vi "MeasurePower.vi"(0 "object in":refnum<class "InstrumentBase.lvclass">, 5 "error in (no error)":errorcluster) -> (14 "object out":refnum<class "InstrumentBase.lvclass">, 16 "Measured Power":dbl, 17 "Channels array":waveform(dbl)[](array[waveform]), 19 "error out":errorcluster)   [LabVIEW 2019, in "InstrumentBase.lvclass"]
uses:
  InstrumentBase.lvclass
  InstrumentBase.lvclass/InstrumentBase.ctl
  <vilib>/Analysis/baseanly.llb/Mean (DBL).vi
  <vilib>/measure/matone.llb/Extract Single Tone Information 1 Chan.vi
  <vilib>/measure/madcrms.llb/Basic Averaged DC-RMS for 1 Chan.vi
  <vilib>/measure/NI_MAPro.lvlib
  <vilib>/Analysis/NI_AALBase.lvlib
panel:
  out "MeasuredPower4":dbl
  out "MeasuredPower3":dbl
  out "Measured Power 2":dbl
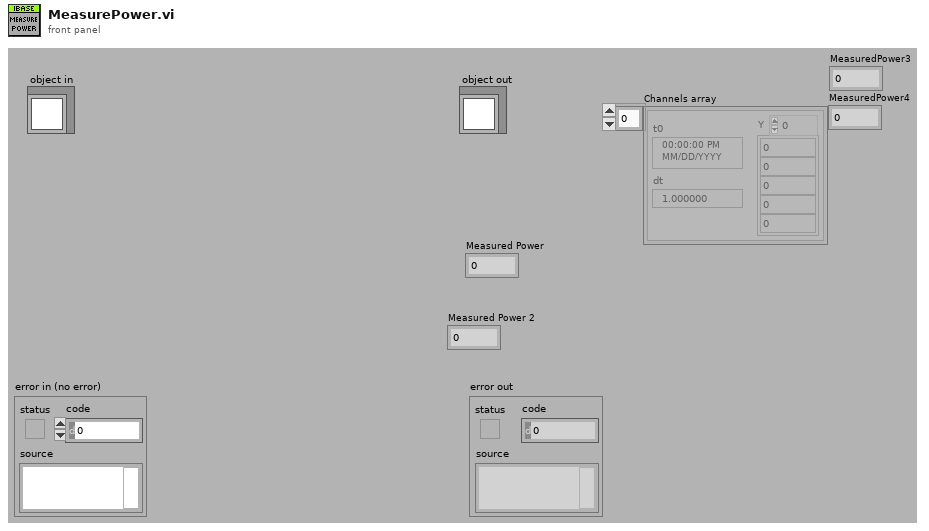
[diagram p1: front panel]
types:
  T1 = enum16{"Rectangular (none)", "Hanning", "Low side lobe"}
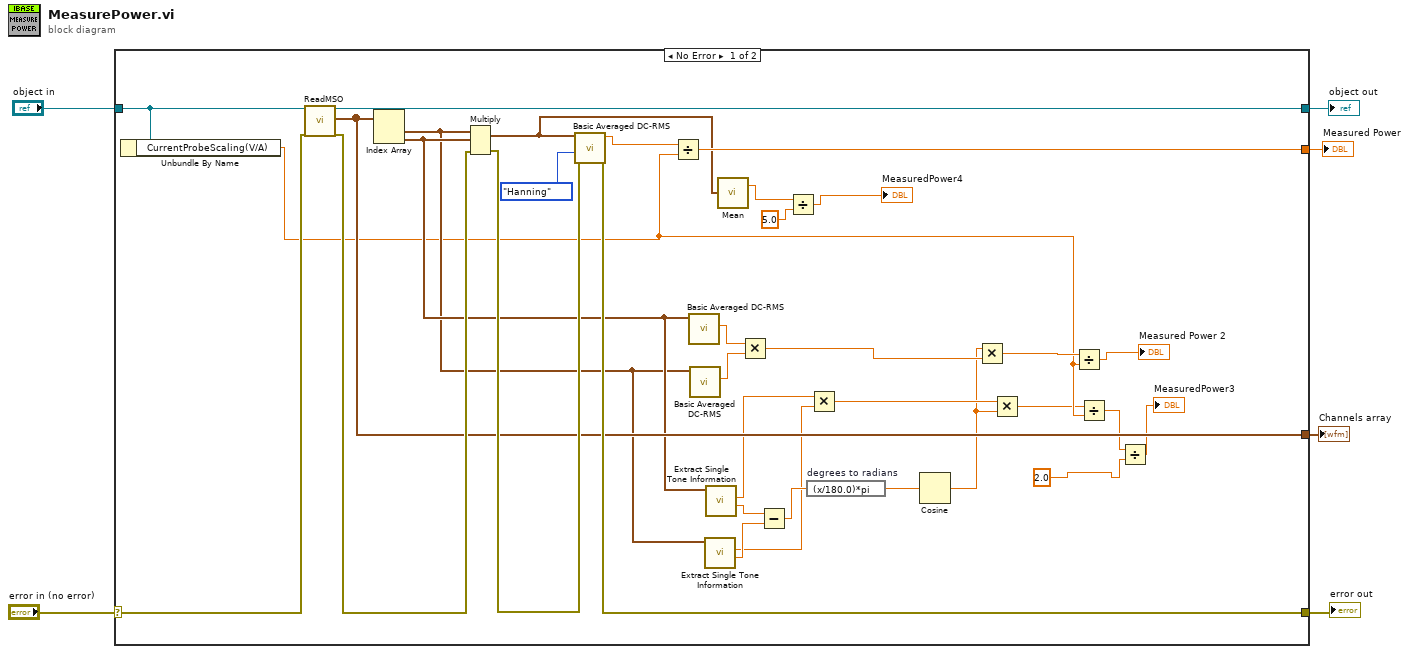
[diagram p0: block diagram]
diagram:
  n1 = case shown="No Error" "error in (no error)" {
    selector: "error in (no error)" -> [w38 w42]
    tunnel: [w35 w42] -> w5
    tunnel: [w40 w41] -> w3
    tunnel: "object in" -> [w33 w41]
    tunnel: [w39 _] -> w2
    tunnel: [w34 _] -> w1
    frame No Error {
      n2 = Unbundle By Name(w33) -> ("CurrentProbeScaling(V/A)"=w16:dbl)
      n3 = call-dynamic "ReadMSO.vi"("object in"=w33, "error in (no error)"=w38) -> ("object out"=w40:refnum<class "InstrumentBase.lvclass">, "Channels array"=w34:waveform(dbl)[], "error out"=w37:errorcluster)  [unwired: 15 in]
      n4 = Index Array(array=w34) -> (element #1=w30:waveform(dbl), element #2=w31:waveform(dbl))  [unwired: 2 in]
      n5 = Multiply(1:w31, 2:w30, 4:w37) -> (0:w11:waveform(dbl), 3:w36:errorcluster)
      n6 = call-poly <vilib>:"Basic Averaged DC-RMS.vi"("error in (no error)"=w36, "window"=T1."Hanning", "signal in"=w11) -> ("error out"=w35:errorcluster, "DC value"=w12:dbl)  [unwired: 5 in, 2 out]
      n7 = Divide(x=w12, y=w16) -> (x/y=w39:dbl)
      n8 = call-poly <vilib>:"Basic Averaged DC-RMS.vi"("signal in"=w31) -> ("RMS value"=w20:dbl)  [unwired: 7 in, 3 out]
      n9 = call-poly <vilib>:"Basic Averaged DC-RMS.vi"("signal in"=w30) -> ("RMS value"=w19:dbl)  [unwired: 7 in, 3 out]
      n10 = call-poly <vilib>:"Extract Single Tone Information.vi"("time signal in"=w30) -> ("detected phase (deg)"=w28:dbl, "detected amplitude"=w24:dbl)  [unwired: 5 in, 4 out]
      n11 = call-poly <vilib>:"Extract Single Tone Information.vi"("time signal in"=w31) -> ("detected phase (deg)"=w29:dbl, "detected amplitude"=w23:dbl)  [unwired: 5 in, 4 out]
      n12 = call-poly <vilib>:"Mean.vi"("X"=w11) -> ("mean"=w10:dbl)  [unwired: 1 out]
      n13 = Multiply(x=w20, y=w19) -> (x*y=w25:dbl)
      n14 = Subtract(x=w29, y=w28) -> (x-y=w27:dbl)
      n15 = Divide(x=w10, y=5.0) -> (x/y=→"MeasuredPower4":dbl)
      n16 = expression code="(x/180.0)*pi" "degrees to radians"(w27) -> (w26:dbl)
      n17 = Multiply(x=w23, y=w24) -> (x*y=w22:dbl)
      n18 = Cosine(x=w26) -> (cos(x)=w21:dbl)
      n19 = Multiply(x=w21, y=w25) -> (x*y=w18:dbl)
      n20 = Multiply(x=w22, y=w21) -> (x*y=w15:dbl)
      n21 = Divide(x=w18, y=w16) -> (x/y=→"Measured Power 2":dbl)
      n22 = Divide(x=w15, y=w16) -> (x/y=w14:dbl)
      n23 = Divide(x=w14, y=2.0 ("x")) -> (x/y=→"MeasuredPower3":dbl)
    }
    frame Error {
    }
  }
  "error out" <- w5
  "object out" <- w3
  "Measured Power" <- w2
  "Channels array" <- w1
